vi "Hardware - NI 9754-2 (ESTTL) Host.vi"() -> ()   [LabVIEW 2015, in "ECS-Host.lvlib"]
uses:
  ECS-Host.lvlib
panel:
  in  "DisableOnCrit":bool caption="Disable On Crit?"
  out "FPGAInterfaceError":bool
  out "_Function List":string[](array[string])
  in  "_Restrike Enable":bool[](array[boolean])
  in  "ChannelRestrikeEnable":u8
  in  "_Ch Enable":bool[](array[boolean])
  out "_Ch List":string[](array[string])
  in  "Restrike3Enable":bool
  in  "Restrike2Enable":bool
  in  "Restrike1Enable":bool
  in  "Restrike3Dwell":sgl=3.0 caption="[]"
  in  "Restrike2Dwell":sgl=3.0 caption="[]"
  in  "Restrike1Dwell":sgl=3.0 caption="[]"
  in  "Delay3":sgl=3.0 caption="[]"
  in  "Delay2":sgl=3.0 caption="[]"
  in  "Ch8Enable":bool
  in  "Ch7Enable":bool
  in  "Ch6Enable":bool
  in  "Ch5Enable":bool
  in  "Ch4Enable":bool
  in  "Ch3Enable":bool
  in  "Ch2Enable":bool
  in  "Ch1Enable":bool
  in  "WindowEnd":sgl caption="[DBTDC]"
  in  "WindowStart":sgl caption="[DBTDC]"
  in  "Delay1":sgl=3.0 caption="[]"
  in  "MainMaxDwell":sgl=20.0 caption="[]"
  # "Enable"
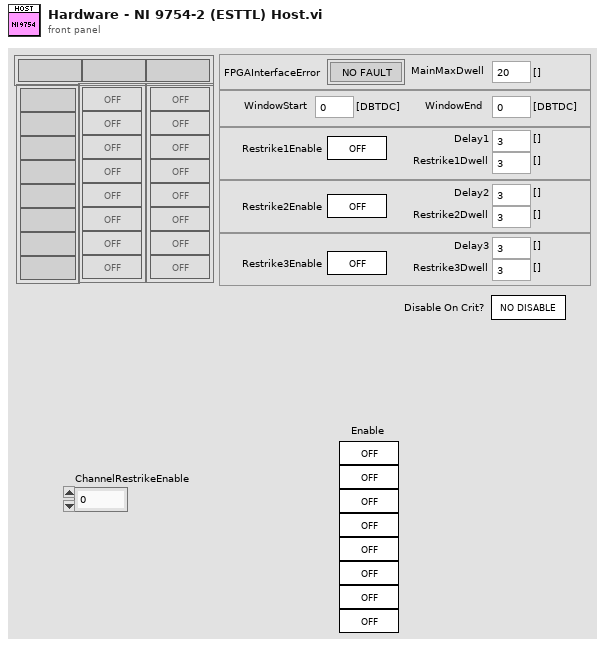
[diagram p1: front panel]
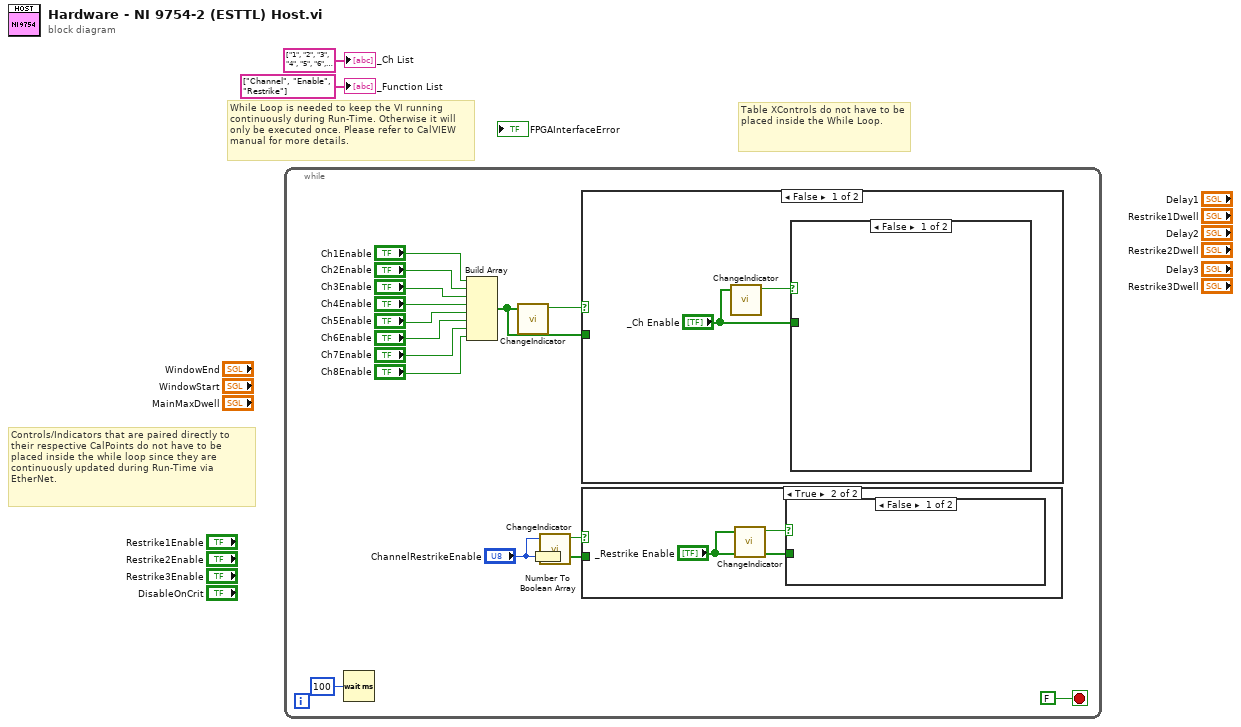
[diagram p0: block diagram]
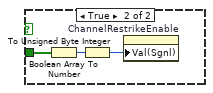
[diagram p3: hidden frame]
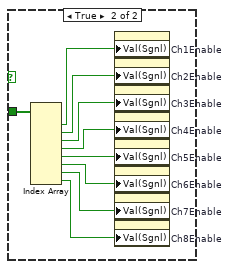
[diagram p4: hidden frame]
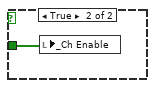
[diagram p5: hidden frame]
diagram:
  # "Table XControls do not have to be placed inside the While Loop."
  # "While Loop is needed to keep the VI running\ncontinuously during Run-Time. Otherwise it will only be executed once. Please refer to CalVIEW manual for more details."
  # "Controls/Indicators that are paired directly to their respective CalPoints do not have to be placed inside the while loop since they are continuously updated during Run-Time via EtherNet."
  n1 = while {
    stop <- FALSE stop-if-true
    n2 = Wait (ms)(milliseconds to wait=u32 100 ("millisecondstowait")) -> ()  [unwired: 1 out]
    n3 = Build Array("Ch1Enable", "Ch2Enable", "Ch3Enable", "Ch4Enable", "Ch5Enable", "Ch6Enable", "Ch7Enable", "Ch8Enable") -> (w6:bool[])
    n4 = call "ChangeIndicator.vi"("Input"=w6) -> ("Change"=w7:bool)  [unwired: 9 in]
    n5 = Number To Boolean Array(number="ChannelRestrikeEnable") -> (Boolean array=w5:bool[])
    n6 = call "ChangeIndicator.vi"("Input"="ChannelRestrikeEnable") -> ("Change"=w4:bool)  [unwired: 9 in]
    n7 = case shown="False" w7 {
      tunnel: w6 -> [_ w34]
      frame False {
        n8 = call "ChangeIndicator.vi"("Input"="_Ch Enable") -> ("Change"=w24:bool)  [unwired: 9 in]
        n9 = case shown="False" w24 {
          tunnel: "_Ch Enable" -> [_ w33]
          frame False {
          }
          frame True {
            n10 = Index Array(array=w33) -> (element #1=w32:bool, element #2=w31:bool, element #3=w30:bool, element #4=w29:bool, element #5=w28:bool, element #6=w27:bool, element #7=w26:bool, element #8=w25:bool)  [unwired: 8 in]
            n11 = property on="Ch1Enable" class="Bool (strict)"("Val(Sgnl)"=w32) -> ()  [unwired: 2 in, 2 out]
            n12 = property on="Ch2Enable" class="Bool (strict)"("Val(Sgnl)"=w31) -> ()  [unwired: 2 in, 2 out]
            n13 = property on="Ch3Enable" class="Bool (strict)"("Val(Sgnl)"=w30) -> ()  [unwired: 2 in, 2 out]
            n14 = property on="Ch4Enable" class="Bool (strict)"("Val(Sgnl)"=w29) -> ()  [unwired: 2 in, 2 out]
            n15 = property on="Ch5Enable" class="Bool (strict)"("Val(Sgnl)"=w28) -> ()  [unwired: 2 in, 2 out]
            n16 = property on="Ch6Enable" class="Bool (strict)"("Val(Sgnl)"=w27) -> ()  [unwired: 2 in, 2 out]
            n17 = property on="Ch7Enable" class="Bool (strict)"("Val(Sgnl)"=w26) -> ()  [unwired: 2 in, 2 out]
            n18 = property on="Ch8Enable" class="Bool (strict)"("Val(Sgnl)"=w25) -> ()  [unwired: 2 in, 2 out]
          }
        }
      }
      frame True {
        n19 = local write "_Ch Enable"(w34) -> ()
      }
    }
    n20 = case shown="True" w4 {
      tunnel: w5 -> [_ _]
      frame False {
      }
      frame True {
        n21 = call "ChangeIndicator.vi"("Input"="_Restrike Enable") -> ("Change"=w19:bool)  [unwired: 9 in]
        n22 = case shown="False" w19 {
          tunnel: "_Restrike Enable" -> [_ w21]
          frame False {
          }
          frame True {
            n23 = Boolean Array To Number(Boolean array=w21) -> (number=w22:u32)
            n24 = To Unsigned Byte Integer(number=w22) -> (unsigned 8bit integer=w20:u8)
            n25 = property on="ChannelRestrikeEnable" class="DigNum (strict)"("Val(Sgnl)"=w20) -> ()  [unwired: 2 in, 2 out]
          }
        }
      }
    }
  }
  "_Ch List" <- string[] ["1", "2", "3", "4", "5", "6", "7", "8"] ("_Ch List")
  "_Function List" <- string[] ["Channel", "Enable", "Restrike"] ("_Function List")
